vi "Get_Variable_Name.vi"(4 "Data":variant) -> (1 "Data Label Name":string)   [LabVIEW 2011]
uses:
  <vilib>/regexp/Match Regular Expression.xnode
panel:
  out "xml string":string
  out "Label.TextByProperty":string
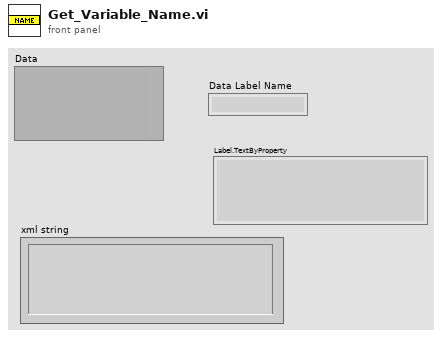
[diagram p1: front panel]
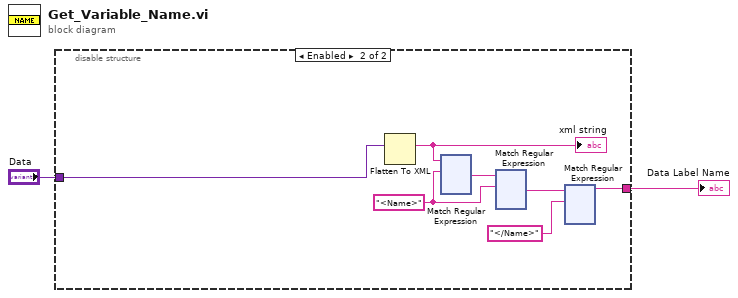
[diagram p0: block diagram]
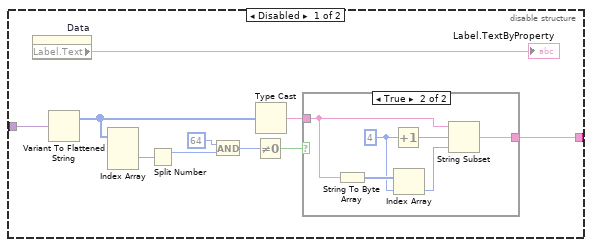
[diagram p2: hidden frame]
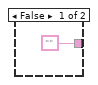
[diagram p3: hidden frame]
diagram:
  n1 = disable-structure shown="Enabled" {
    disable-tunnel: "Data" -> [w4 w21]
    disable-tunnel: [w3 w20] -> w1
    frame Disabled {
      n2 = property on="Data" class="LVVar"() -> ("Label.Text"=→"Label.TextByProperty":string)  [unwired: 2 in, 2 out]
      n3 = Variant To Flattened String(Variant=w4) -> (1:w10:i16[])  [unwired: 1 out]
      n4 = Index Array(array=w10) -> (element #2=w9:i16)  [unwired: 3 in, 2 out]
      n5 = Split Number(x=w9) -> (hi(x)=w8:u8)  [unwired: 1 out]
      n6 = And(x=64, y=w8) -> (x .and. y?=w12:i32)
      n7 = Not Equal To 0?(x=w12) -> (x != 0?=w6:bool)
      n8 = Type Cast(x=w10) -> (*(type *) &x=w7:string)  [unwired: 1 in]
      n9 = case shown="True" w6 {
        tunnel: w7 -> [_ w18]
        tunnel: ["" w14] -> w3
        frame False {
        }
        frame True {
          w15 = 4 ("x")
          n10 = String To Byte Array(string=w18) -> (unsigned byte array=w19:u8[])
          n11 = Increment(x=w15) -> (x+1=w17:i32)
          n12 = Index Array(array=w19, index=w15) -> (element=w16:u8)
          n13 = String Subset(string=w18, offset (0)=w17, length (rest)=w16) -> (substring=w14:string)
        }
      }
    }
    frame Enabled {
      w24 = "<Name>" ("regular expression")
      n14 = Flatten To XML(anything=w21) -> (xml string=w22:string)
      "xml string" <- w22
      n15 = xnode "Match Regular Expression"("input string"=w22, "regular expression"=w24) -> ("after match"=w23:string)  [unwired: 4 in, 4 out]
      n16 = xnode "Match Regular Expression"("input string"=w23, "regular expression"=w24) -> ("after match"=w25:string)  [unwired: 4 in, 4 out]
      n17 = xnode "Match Regular Expression"("input string"=w25, "regular expression"="</Name>") -> ("before match"=w20:string)  [unwired: 4 in, 4 out]
    }
  }
  "Data Label Name" <- w1
